vi "calucation.vi"(9 "String 2":string, 10 "String":string, 11 "String 3":string) -> (3 "String 4":string)   [LabVIEW 2022 SP3]
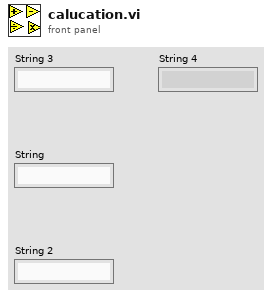
[diagram p1: front panel]
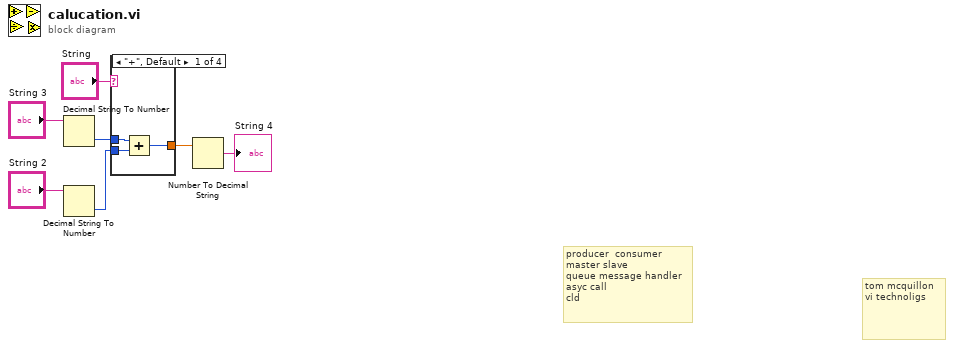
[diagram p0: block diagram]
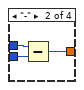
[diagram p2: hidden frame]
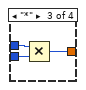
[diagram p3: hidden frame]
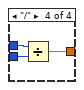
[diagram p4: hidden frame]
diagram:
  # "tom mcquillon\nvi technoligs"
  # "producer  consumer\nmaster slave\nqueue message handler\nasyc call\ncld"
  n1 = Decimal String To Number(string="String 3") -> (number=w2:i32)  [unwired: 2 in, 1 out]
  n2 = Decimal String To Number(string="String 2") -> (number=w4:i32)  [unwired: 2 in, 1 out]
  n3 = case shown="\"+\", Default" "String" {
    tunnel: [w10 w12 w16 w19] -> w3
    tunnel: w2 -> [w9 w13 w15 w18]
    tunnel: w4 -> [w8 w11 w14 w17]
    frame "+", Default {
      n4 = Add(x=w9, y=w8) -> (x+y=w10:i32)
    }
    frame "-" {
      n5 = Subtract(x=w13, y=w11) -> (x-y=w12:i32)
    }
    frame "*" {
      n6 = Multiply(x=w15, y=w14) -> (x*y=w16:i32)
    }
    frame "/" {
      n7 = Divide(x=w18, y=w17) -> (x/y=w19:dbl)
    }
  }
  n8 = Number To Decimal String(number=w3) -> (decimal integer string=→"String 4":string)  [unwired: 1 in]
